vi "总磷质控流程.vi"(6 "队列输入TP":refnum<queue>, 9 "总磷":bool, 10 "总磷量程切换":enum32{"H", "L", "AUTO"}(ring)=enum."AUTO") -> (3 "布尔":bool)   [LabVIEW 2016, in "质控单元.lvlib"]
panel:
  out "总磷中断报警":bool
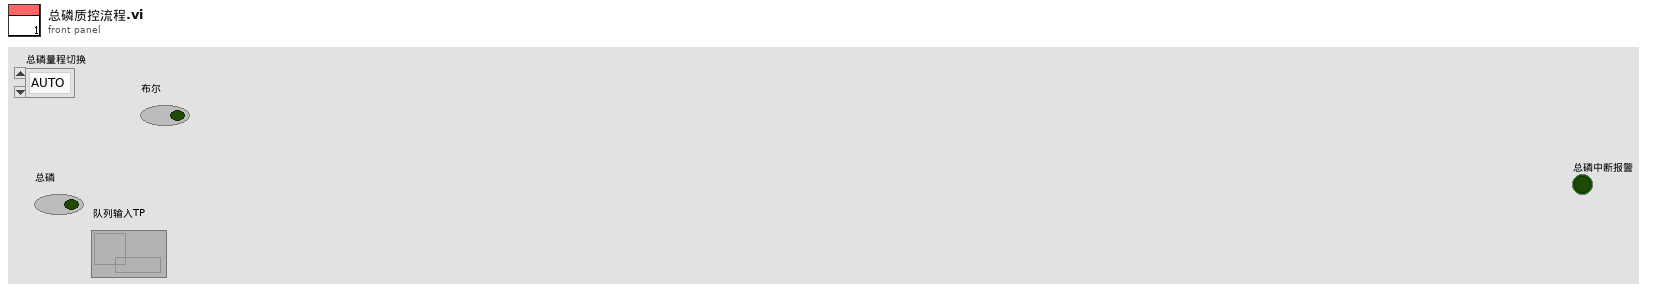
[diagram p1: front panel]
types:
  T1 = enum16{"待机", "启动氨氮水样", "氨氮测量中", "启动氨氮加标", "启动氨氮加标回收", "氨氮加标回收测量中", "启动总氮水样", "总氮测量中", "启动总氮加标", "启动总氮加标回收", "总氮加标回收测量中", "启动总磷水样", "总磷水样测量中", "启动总磷加标", "启动总磷加标回收", "总磷加标回收测量中", "结束"}
  T2 = cluster{"站号":u16, "量程切换":enum32{"H", "L", "AUTO"}, "控制命令":enum16{"启动测量", "标样核查", "零点核查", "跨度核查", "空白测试", "平行样测试", "加标回收", "空白校准", "标样校准", "初始化（清洗）", "停止测试", "仪器重启", "校时", "模式设置", "测量间隔设置"}, "模式设置":enum16{"待机", "连续模式", "周期模式", "定点模式", "受控模式", "手动模式"}, "测量间隔":u16}
  T3 = cluster{"时间标识":timestamp, "设备":string, "日志信息":string}
  T4 = cluster{"系统时间":timestamp, "工作状态":enum16{"空闲", "水样测试", "标样核查", "零点核查", "跨度核查", "空白测试", "平行样测试", "加标回收", "空白校准", "标样校准", "初始化（清洗）"}, "测量模式":enum16{"待机", "连续模式", "周期模式", "定点模式", "受控模式", "手动模式"}, "告警代码":enum16{"无告警", "缺试剂告警", "缺水样告警", "缺蒸馏水告警", "缺标液告警", "仪表漏液告警", "标定异常告警", "超量程告警", "加热异常", "低试剂预警", "超上限告警", "超下限告警", "仪表内部其他异常", "滴定异常告警", "电极异常告警", "量程切换告警", "参数设置告警", "PH电极电位异常", "电导率电极异常", "浊度光度异常", "溶解氧电极异常", "溶解氧光强异常", "温度异常告警", "PH异常告警", "溶解氧异常告警", "电导率异常告警", "浊度异常告警", "叶绿素异常告警", "藻密度异常告警", "蓝绿藻异常告警", "ORP异常告警", "氨氮异常告警", "清洁刷异常告警", "SD卡异常告警", "蓝牙异常告警", "Wifi异常告警", "流程异常告警"}, "故障代码":enum16{"无故障", "电机故障", "温度故障", "通讯故障", "滴定故障"}, "日志代码":u16, "软件版本":u16, "F0":sgl, "F1":sgl, "F2":sgl, "F3":sgl, "T":sgl, "H":sgl, "id":u16, "flowid":u16, "量程":u16, "总磷控温温度1":sgl, "营养盐控温温度2":sgl, "ADC":sgl}
  T5 = enum16{"空闲", "水样测试", "标样核查", "零点核查", "跨度核查", "空白测试", "平行样测试", "加标回收", "空白校准", "标样校准", "初始化（清洗）"}
  T6 = cluster{"因子编码":u32, "单位":u16, "标样参考值":sgl, "水样数据时间":timestamp, "水样实测值":sgl, "水样数据标识":string, "标样数据时间":timestamp, "标样实测值":sgl, "标样数据标识":string, "空白数据时间":timestamp, "空白实测值":sgl, "空白数据标识":string, "零点核查数据时间":timestamp, "零点核查实测值":sgl, "零点核查数据标识":string, "跨度核查数据时间":timestamp, "跨度核查实测值":sgl, "跨度核查数据标识":string, "加标回收数据时间":timestamp, "加标回收实测值":sgl, "加标回收数据标识":string, "平行样数据时间":timestamp, "平行样实测值":sgl, "平行样数据标识":string}
  T7 = cluster{"量程":dbl, "检出限":dbl, "加标前水样浓度":dbl, "加标后水样浓度":dbl, "加标水杯定容体积":dbl, "加标母液浓度":dbl, "加标体积":dbl, "加标回收率":dbl}
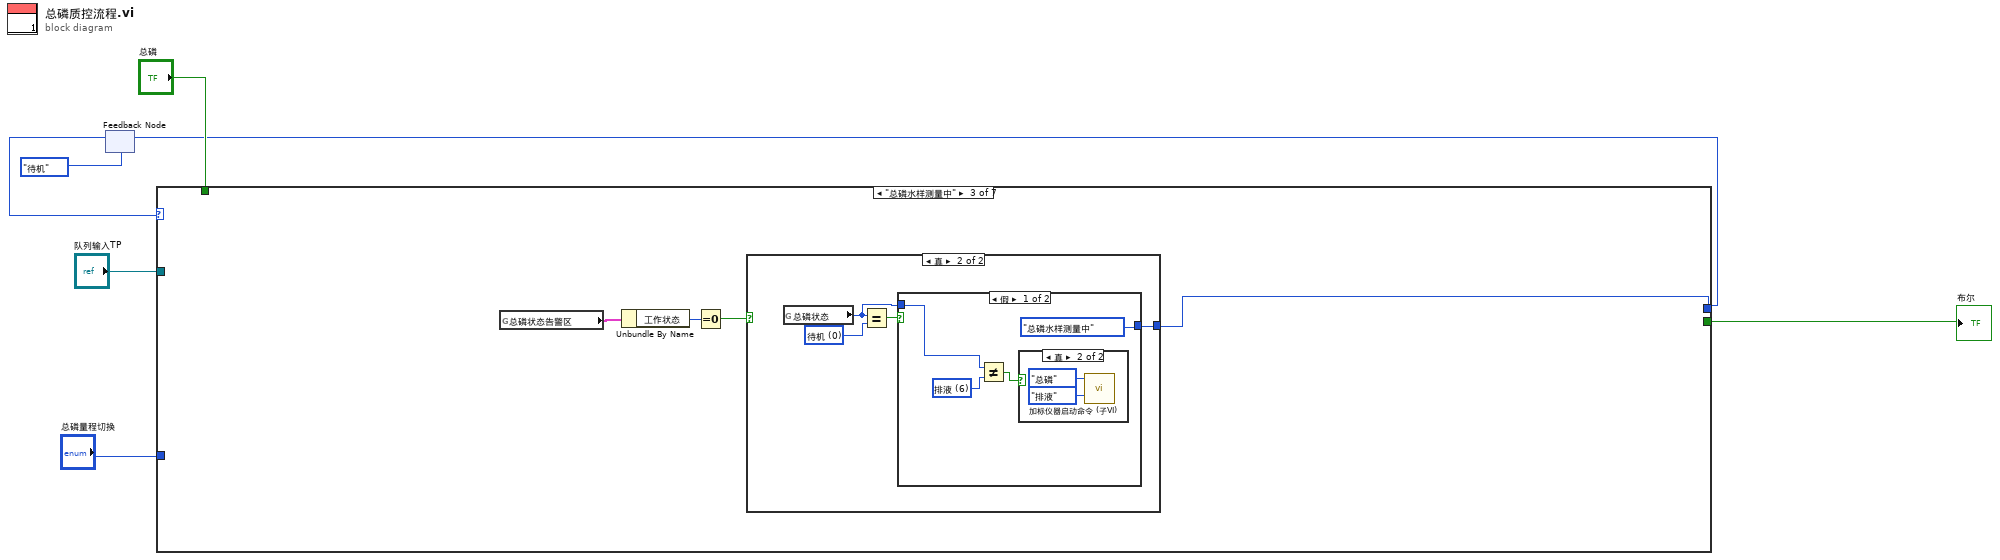
[diagram p0: block diagram]
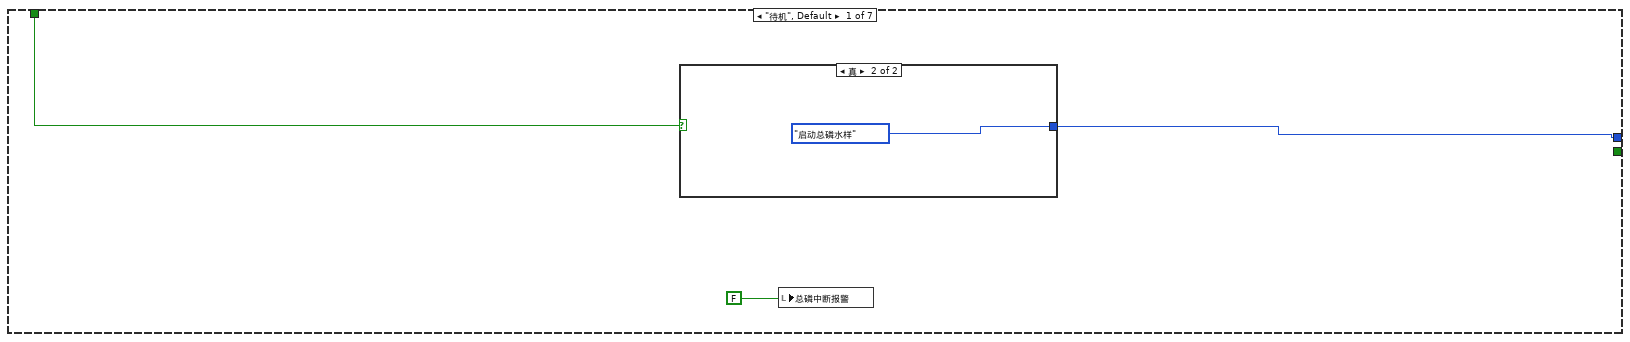
[diagram p2: hidden frame]
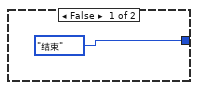
[diagram p3: hidden frame]
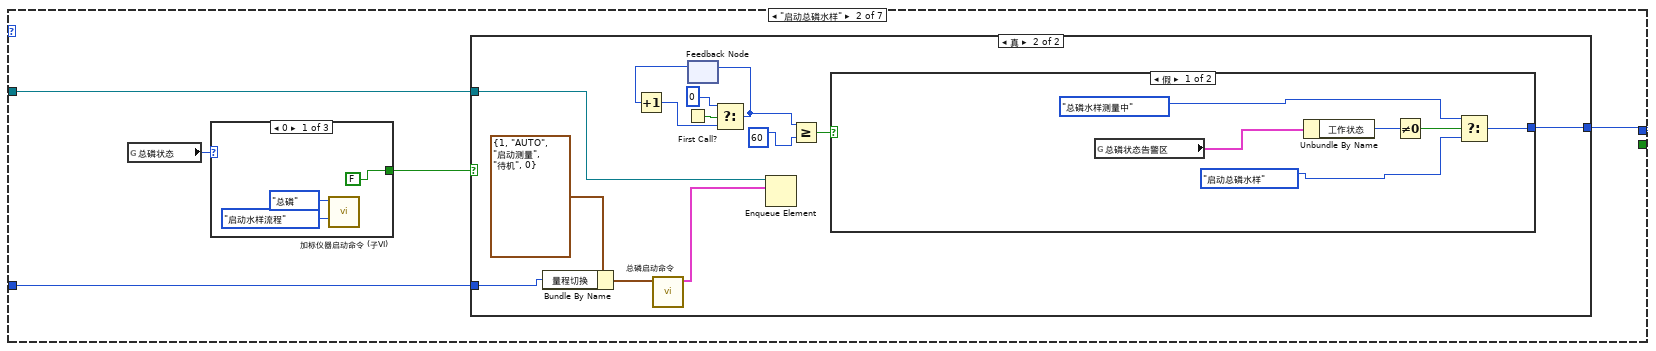
[diagram p4: hidden frame]
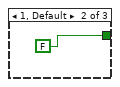
[diagram p5: hidden frame]
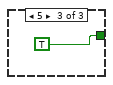
[diagram p6: hidden frame]
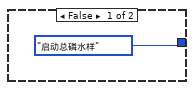
[diagram p7: hidden frame]
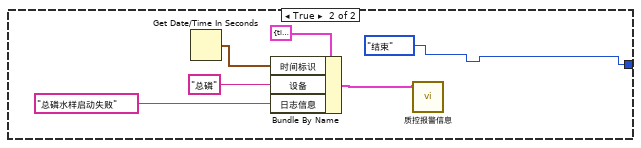
[diagram p8: hidden frame]
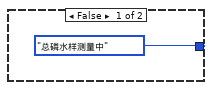
[diagram p9: hidden frame]
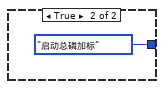
[diagram p11: hidden frame]
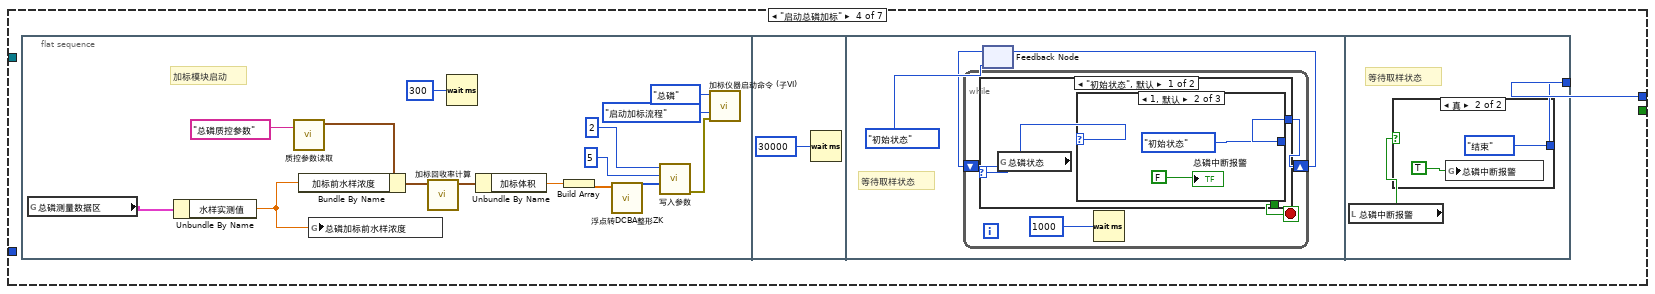
[diagram p12: hidden frame]
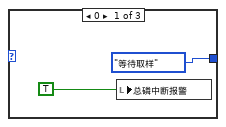
[diagram p13: hidden frame]
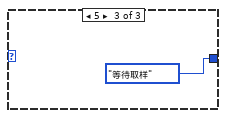
[diagram p14: hidden frame]
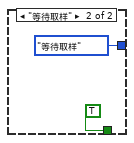
[diagram p15: hidden frame]
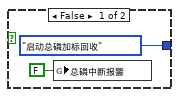
[diagram p16: hidden frame]
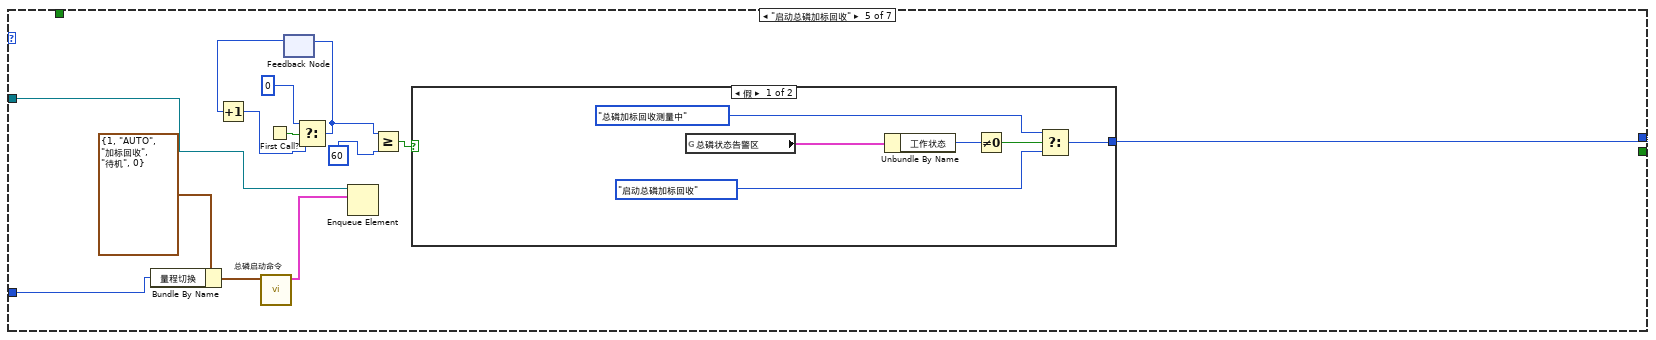
[diagram p17: hidden frame]
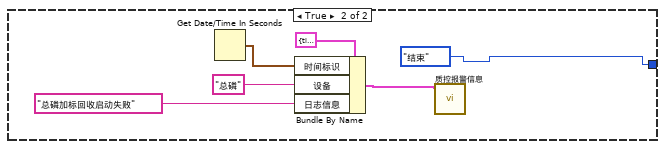
[diagram p18: hidden frame]
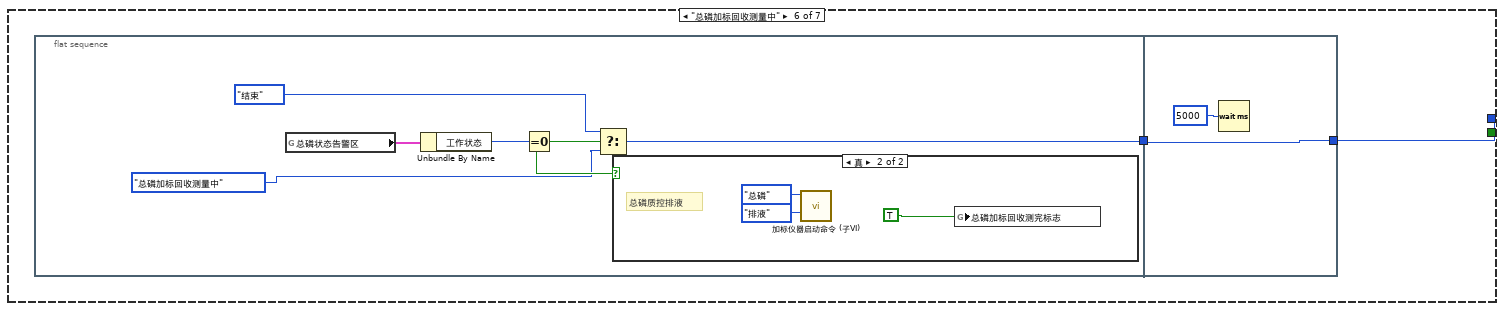
[diagram p19: hidden frame]
diagram:
  n1 = feedback #1(T1."待机") -> (w5:T1)
  n2 = case shown="\"总磷水样测量中\"" w5 {
    tunnel: [w10 w17 w49 w65 w109 w129 T1."结束"] -> w3
    tunnel: [_ _ _ _ _ _ TRUE] -> w6
    tunnel: "总磷" -> [w9 _ _ _ _ _ _]
    tunnel: "队列输入TP" -> [_ w16 _ _ w108 _ _]
    tunnel: "总磷量程切换" -> [_ w15 _ _ w104 _ _]
    frame "待机", Default {
      n3 = case shown="真" w9 {
        tunnel: [T1."结束" T1."启动总磷水样"] -> w10
        frame False {
        }
        frame True {
        }
      }
      n4 = local write "总磷中断报警"(FALSE ("氨氮中断报警")) -> ()
    }
    frame "启动总磷水样" {
      n5 = global read "加标回收状态全局变量.vi" "总磷状态"() -> (w14:u16)
      n6 = case shown="0" w14 {
        tunnel: [FALSE ("s") FALSE ("s") TRUE ("s")] -> w13
        frame 0 {
          n7 = call "加标仪器启动命令 (子VI).vi"("启动命令"=enum16{"启动水样流程", "启动加标流程", "排液", "停止"}."启动水样流程", "仪器"=enum16{"", "氨氮", "总磷", "总氮", "CODMn", "CODCr"}."总磷") -> ()  [unwired: 9 in, 1 out]
        }
        frame 1, Default {
        }
        frame 5 {
        }
      }
      n8 = case shown="真" w13 {
        tunnel: [T1."启动总磷水样" w36] -> w17
        tunnel: w16 -> [_ w25]
        tunnel: w15 -> [_ w24]
        frame False {
        }
        frame True {
          n9 = Bundle By Name(cluster=T2 {"站号"=1, "量程切换"=enum."AUTO", "控制命令"=enum."启动测量", "模式设置"=enum."待机", "测量间隔"=0} ("参数"), "量程切换"=w24) -> (w28:T2)
          n10 = call "总磷启动命令.vi"("参数"=w28) -> ("启动命令"=w26:cluster{"命令":string, "data":variant})  [unwired: 10 in]
          n11 = First Call?() -> (First Call?: T/F=w34:bool)
          n12 = feedback #2() -> (w33:i32)  [unwired: 1 in]
          n13 = Increment(x=w33) -> (x+1=w29:i32)
          n14 = Select(t=0, s=w34, f=w29) -> (s? t:f=w32:i32)
          n15 = feedback-in #2(w32) -> ()
          n16 = Enqueue Element(queue=w25, element=w26) -> ()  [unwired: 2 in, 3 out]
          n17 = Greater Or Equal?(x=w32, y=60) -> (x >= y?=w30:bool)
          n18 = case shown="假" w30 {
            tunnel: [w40 T1."结束"] -> w36
            frame False {
              n19 = global read "与总磷交互全局.vi" "总磷状态告警区"() -> (w37:T4)
              n20 = Unbundle By Name(w37) -> ("工作状态"=w42:T5)
              n21 = Not Equal To 0?(x=w42) -> (x != 0?=w41:bool)
              n22 = Select(t=T1."总磷水样测量中", s=w41, f=T1."启动总磷水样") -> (s? t:f=w40:T1)
            }
            frame True {
              n23 = Get Date/Time In Seconds() -> (seconds since 1Jan1904=w48:timestamp)
              n24 = Bundle By Name(cluster=T3 {"时间标识"=timestamp(0 s since 1904-01-01), "设备"="", "日志信息"=""} ("data in"), "时间标识"=w48, "设备"="总磷", "日志信息"="总磷水样启动失败") -> (w43:T3)
              n25 = call "质控报警信息.vi"("data in"=w43) -> ()  [unwired: 10 in, 1 out]
            }
          }
        }
      }
    }
    frame "总磷水样测量中" {
      n26 = global read "与总磷交互全局.vi" "总磷状态告警区"() -> (w52:T4)
      n27 = Unbundle By Name(w52) -> ("工作状态"=w50:T5)
      n28 = Equal To 0?(x=w50) -> (x = 0?=w51:bool)
      n29 = case shown="真" w51 {
        tunnel: [T1."总磷水样测量中" w55] -> w49
        frame False {
        }
        frame True {
          w57 = u16 0 items=["待机", "润洗", "进样", "进样完成", "柱塞泵加标", "等待取液", "排液"] ("氨氮状态")
          n30 = global read "加标回收状态全局变量.vi" "总磷状态"() -> (w54:u16)
          n31 = Equal?(x=w54, y=w57) -> (x = y?=w56:bool)
          n32 = case shown="假" w56 {
            tunnel: [T1."总磷水样测量中" T1."启动总磷加标"] -> w55
            tunnel: w54 -> [w59 _]
            frame False {
              w60 = u16 6 items=["待机", "润洗", "进样", "进样完成", "柱塞泵加标", "等待取液", "排液"] ("氨氮状态")
              n33 = Not Equal?(x=w59, y=w60) -> (x != y?=w58:bool)
              n34 = case shown="真" w58 {
                frame False {
                }
                frame True {
                  n35 = call "加标仪器启动命令 (子VI).vi"("启动命令"=enum16{"启动水样流程", "启动加标流程", "排液", "停止"}."排液", "仪器"=enum16{"", "氨氮", "总磷", "总氮", "CODMn", "CODCr"}."总磷") -> ()  [unwired: 9 in, 1 out]
                }
              }
            }
            frame True {
            }
          }
        }
      }
    }
    frame "启动总磷加标" {
      n36 = flat-sequence {
        tunnel: [w99] -> w65
        frame #0 {
          # "加标模块启动"
          n37 = global read "与总磷交互全局.vi" "总磷测量数据区"() -> (w71:T6)
          n38 = Unbundle By Name(w71) -> ("水样实测值"=w73:sgl)
          n39 = call "质控参数读取.vi"("section"="总磷质控参数") -> ("参数"=w78:T7)  [unwired: 9 in, 1 out]
          n40 = Bundle By Name(cluster=w78, "加标前水样浓度"=w73) -> (w79:T7)
          n41 = global write "水样浓度全局.vi" "总磷加标前水样浓度"(w73) -> ()
          n42 = call "加标回收率计算.vi"("参数"=w79) -> ("参数 out"=w77:T7)  [unwired: 10 in]
          n43 = Wait (ms)(milliseconds to wait=u32 300 ("等待时间（毫秒）")) -> ()  [unwired: 1 out]
          n44 = Unbundle By Name(w77) -> ("加标体积"=w74:dbl)
          n45 = Build Array(w74) -> (w70:dbl[])
          n46 = call "浮点转DCBA整形ZK.vi"("浮点数"=w70) -> ("DCBA整形输出"=w69:u16[])  [unwired: 10 in]
          n47 = call "写入参数.vi"("values"=w69, "starting address"=u16 5, "Slave ID"=u16 2 ("value")) -> ("error out"=w66:errorcluster)  [unwired: 8 in]
          n48 = call "加标仪器启动命令 (子VI).vi"("Error in"=w66, "启动命令"=enum16{"启动水样流程", "启动加标流程", "排液", "停止"}."启动加标流程", "仪器"=enum16{"", "氨氮", "总磷", "总氮", "CODMn", "CODCr"}."总磷") -> ()  [unwired: 8 in, 1 out]
        }
        frame #1 {
          n49 = Wait (ms)(milliseconds to wait=u32 30000 ("等待时间（毫秒）")) -> ()  [unwired: 1 out]
        }
        frame #2 {
          # "等待取样状态"
          n50 = feedback #3(enum16{"初始状态", "等待取样"}."初始状态") -> (w83:enum16{"初始状态", "等待取样"})
          n51 = while {
            shift-right: [w87] -> w82
            shift-left: w83 -> [w88]
            stop <- w86 stop-if-true
            n52 = case shown="\"初始状态\", 默认" w88 {
              tunnel: [w90 enum16{"初始状态", "等待取样"}."等待取样"] -> w87
              tunnel: [_ TRUE] -> w86
              frame "初始状态", Default {
                n53 = global read "加标回收状态全局变量.vi" "总磷状态"() -> (w89:u16)
                n54 = case shown="1, 默认" w89 {
                  tunnel: [enum16{"初始状态", "等待取样"}."等待取样" enum16{"初始状态", "等待取样"}."初始状态" enum16{"初始状态", "等待取样"}."等待取样"] -> w90
                  frame 0 {
                    n55 = local write "总磷中断报警"(TRUE ("氨氮中断报警")) -> ()
                  }
                  frame 1, Default {
                    "总磷中断报警" <- FALSE ("总氮中断报警")
                  }
                  frame 5 {
                  }
                }
              }
              frame "等待取样" {
              }
            }
            n56 = Wait (ms)(milliseconds to wait=u32 1000 ("等待时间（毫秒）")) -> ()  [unwired: 1 out]
          }
          n57 = feedback-in #3(w82) -> ()
        }
        frame #3 {
          # "等待取样状态"
          n58 = local read "总磷中断报警"() -> (w98:bool)
          n59 = case shown="真" w98 {
            tunnel: [T1."启动总磷加标回收" T1."结束"] -> w99
            frame False {
              n60 = global write "质控中断报警全局.vi" "总磷中断报警"(FALSE ("总磷中断报警")) -> ()
            }
            frame True {
              n61 = global write "质控中断报警全局.vi" "总磷中断报警"(TRUE ("总磷中断报警")) -> ()
            }
          }
        }
      }
    }
    frame "启动总磷加标回收" {
      n62 = Bundle By Name(cluster=T2 {"站号"=1, "量程切换"=enum."AUTO", "控制命令"=enum."加标回收", "模式设置"=enum."待机", "测量间隔"=0} ("参数"), "量程切换"=w104) -> (w106:T2)
      n63 = call "总磷启动命令.vi"("参数"=w106) -> ("启动命令"=w105:cluster{"命令":string, "data":variant})  [unwired: 10 in]
      n64 = First Call?() -> (First Call?: T/F=w115:bool)
      n65 = feedback #4() -> (w114:i32)  [unwired: 1 in]
      n66 = Increment(x=w114) -> (x+1=w113:i32)
      n67 = Select(t=0, s=w115, f=w113) -> (s? t:f=w112:i32)
      n68 = feedback-in #4(w112) -> ()
      n69 = Enqueue Element(queue=w108, element=w105) -> ()  [unwired: 2 in, 3 out]
      n70 = Greater Or Equal?(x=w112, y=60) -> (x >= y?=w110:bool)
      n71 = case shown="假" w110 {
        tunnel: [w120 T1."结束"] -> w109
        frame False {
          n72 = global read "与总磷交互全局.vi" "总磷状态告警区"() -> (w117:T4)
          n73 = Unbundle By Name(w117) -> ("工作状态"=w122:T5)
          n74 = Not Equal To 0?(x=w122) -> (x != 0?=w121:bool)
          n75 = Select(t=T1."总磷加标回收测量中", s=w121, f=T1."启动总磷加标回收") -> (s? t:f=w120:T1)
        }
        frame True {
          n76 = Get Date/Time In Seconds() -> (seconds since 1Jan1904=w128:timestamp)
          n77 = Bundle By Name(cluster=T3 {"时间标识"=timestamp(0 s since 1904-01-01), "设备"="", "日志信息"=""} ("data in"), "时间标识"=w128, "设备"="总磷", "日志信息"="总磷加标回收启动失败") -> (w123:T3)
          n78 = call "质控报警信息.vi"("data in"=w123) -> ()  [unwired: 10 in, 1 out]
        }
      }
    }
    frame "总磷加标回收测量中" {
      n79 = flat-sequence {
        tunnel: [w135] -> w130
        tunnel: [w141] -> w129
        tunnel: w130 -> [w141]
        frame #0 {
          n80 = global read "与总磷交互全局.vi" "总磷状态告警区"() -> (w131:T4)
          n81 = Unbundle By Name(w131) -> ("工作状态"=w136:T5)
          n82 = Equal To 0?(x=w136) -> (x = 0?=w133:bool)
          n83 = Select(t=T1."结束", s=w133, f=T1."总磷加标回收测量中") -> (s? t:f=w135:T1)
          n84 = case shown="真" w133 {
            frame False {
            }
            frame True {
              # "总磷质控排液"
              n85 = call "加标仪器启动命令 (子VI).vi"("启动命令"=enum16{"启动水样流程", "启动加标流程", "排液", "停止"}."排液", "仪器"=enum16{"", "氨氮", "总磷", "总氮", "CODMn", "CODCr"}."总磷") -> ()  [unwired: 9 in, 1 out]
              n86 = global write "质控测完标志全局 1.vi" "总磷加标回收测完标志"(TRUE) -> ()
            }
          }
        }
        frame #1 {
          n87 = Wait (ms)(milliseconds to wait=u32 5000 ("等待时间（毫秒）")) -> ()  [unwired: 1 out]
        }
      }
    }
    frame "结束" {
    }
  }
  "布尔" <- w6
  n88 = feedback-in #1(w3) -> ()
